vi "Assignment 2.vi"() -> ()   [LabVIEW 2018]
panel:
  out "Current Maximum number":dbl
  out "Current Minimum number":dbl
  out "Current Random number":dbl
  out "Iteration":dbl
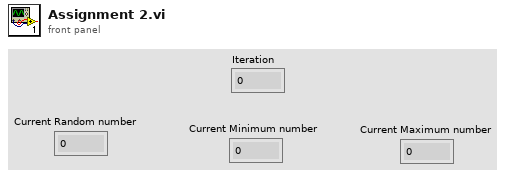
[diagram p1: front panel]
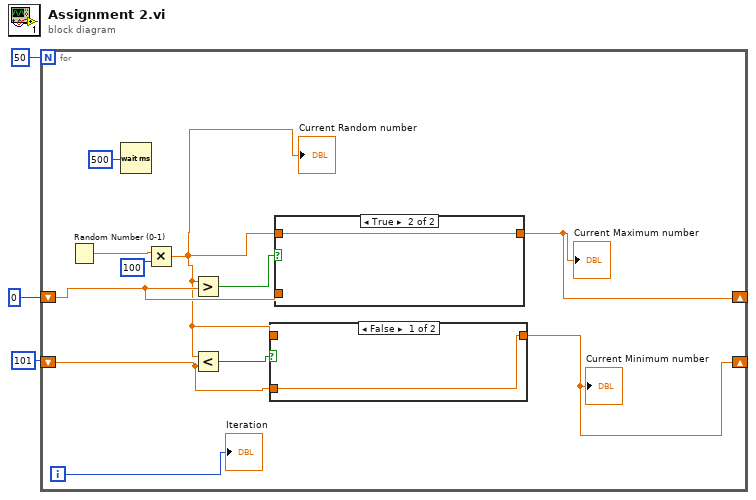
[diagram p0: block diagram]
diagram:
  n1 = for {
    N: 50 -> [_]
    shift-right: [w8] -> _
    shift-left: 0 -> [w9]
    shift-right: [w4] -> _
    shift-left: 101 -> [w5]
    i -> [w11]
    n2 = Random Number (0-1)() -> (number: 0 to 1=w13:dbl)
    n3 = Wait (ms)(milliseconds to wait=500) -> ()  [unwired: 1 out]
    n4 = Multiply(x=w13, y=100) -> (x*y=w6:dbl)
    "Current Random number" <- w6
    n5 = Greater?(x=w6, y=w9) -> (0:w10:bool)
    n6 = Less?(x=w6, y=w5) -> (x < y?=w7:bool)
    n7 = case shown="False" w7 {
      tunnel: w6 -> [_ w16]
      tunnel: w5 -> [w15 _]
      tunnel: [w15 w16] -> w4
      frame False {
      }
      frame True {
      }
    }
    "Current Minimum number" <- w4
    n8 = case shown="True" w10 {
      tunnel: w6 -> [_ w18]
      tunnel: w9 -> [w17 _]
      tunnel: [w17 w18] -> w8
      frame False {
      }
      frame True {
      }
    }
    "Current Maximum number" <- w8
    "Iteration" <- w11
  }
